vi "Snap.vi"(5 "State In":T1, 7 "Low/Tiny":bool, 8 "error in (no error)":errorcluster, 10 "IMAQ Refs Dani":T3) -> (0 "error out":errorcluster, 1 "Objects":T2[](array[typedef]) {"Aspect Ratio" format="%.2f"; "Orientation" format="%.2f"; "Area" format="%.2f"; "Object Center"."Y" format="%.2f"; "Object Center"."X" format="%.2f"})   [LabVIEW 2015]
uses:
  TypeDefs Host/IMAQ Refs.ctl
  <vilib>/vision/Image Controls.llb/IMAQ Image.ctl
  TypeDefs Host/Object Info.ctl
  TypeDefs Host/States.ctl
  TypeDefs Host/Counter FGV Enum.ctl
  TypeDefs Host/Open Audio FGV Enum.ctl
  <vilib>/vision/NI_Vision_Development_Module.lvlib
panel:
  out "Elapsed time (ms)":u32
  out "Number of Objects":i32
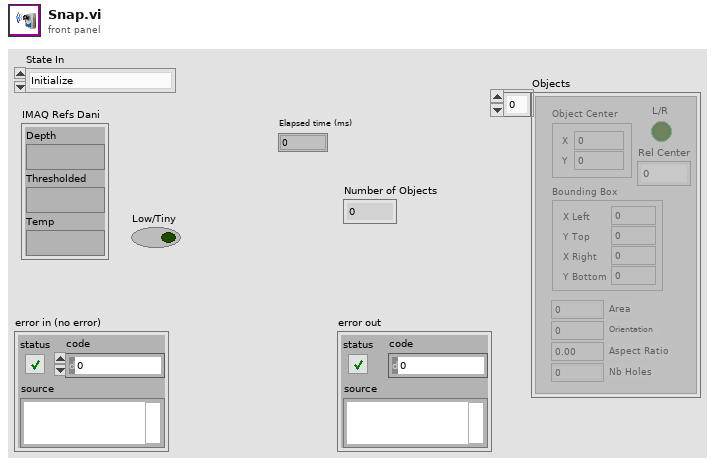
[diagram p1: front panel]
types:
  T1 = typedef "States.ctl" = enum16{"Initialize", "Calibrate", "Create", "Settings", "Shutdown"}
  T2 = typedef "Object Info.ctl" = cluster{"Object Center":cluster{"X":u16, "Y":u16}, "Bounding Box":cluster{"X Left":u16, "Y Top":u16, "X Right":u16, "Y Bottom":u16}, "Area":u16, "Orientation":u16, "Aspect Ratio":sgl, "Nb Holes":u16, "L/R":bool, "Rel Center":u16}
  T3 = typedef "IMAQ Refs.ctl" = cluster{"Thresholded":T4, "Temp":T4, "Depth":T4}
  T4 = typedef "IMAQ Image.ctl" = refnum<image>
  T5 = typedef "Counter FGV Enum.ctl" = enum16{"Get Count", "Set Count"}
  T6 = cluster{"Objects":u16, "Threshold":i32, "Reject Border":bool, "Fill Holes":bool, "Min Object Size":bool, "Min Size":i32, "Max Object Size":bool, "Max Size":i32, "Show Search Area":bool, "Show Center":bool, "Show Bounding Box":bool}
  T7 = typedef "Open Audio FGV Enum.ctl" = enum16{"Get", "Set"}
  T8 = typedef "IMAQ Rectangle" = cluster{"Left":i32, "Top":i32, "Right":i32, "Bottom":i32, "Rotation":dbl}
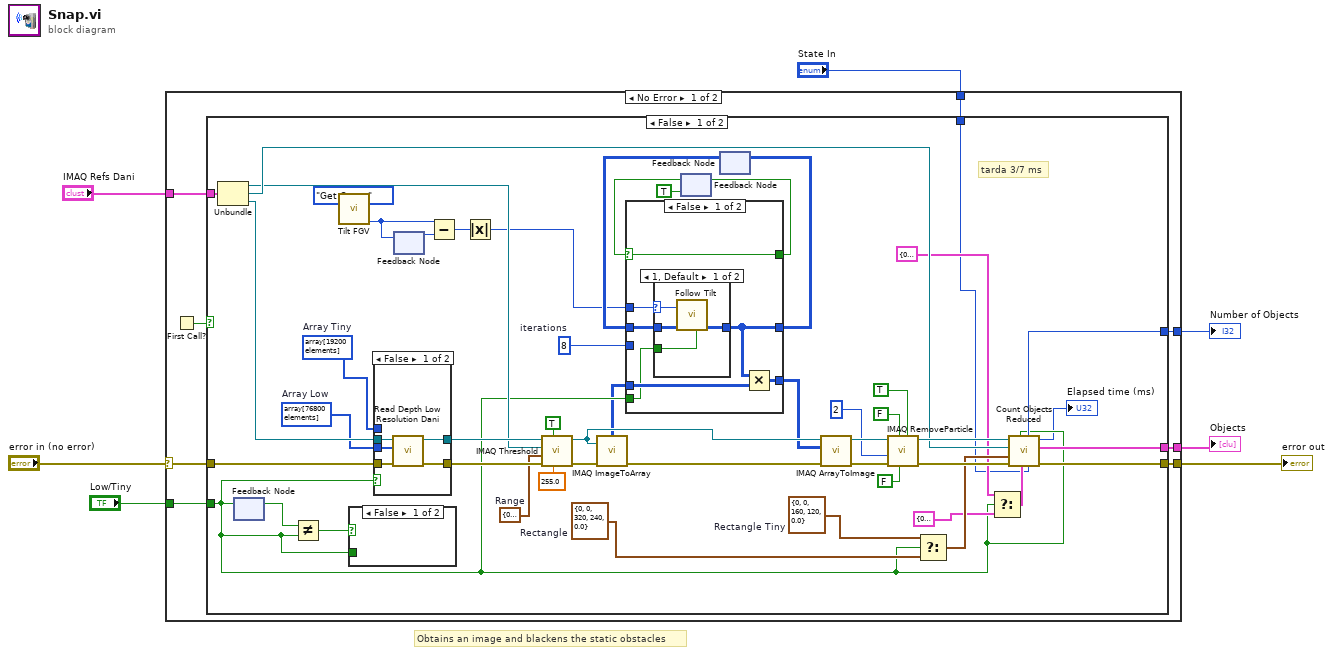
[diagram p0: block diagram]
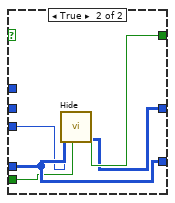
[diagram p3: hidden frame]
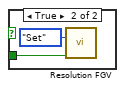
[diagram p4: hidden frame]
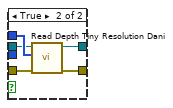
[diagram p5: hidden frame]
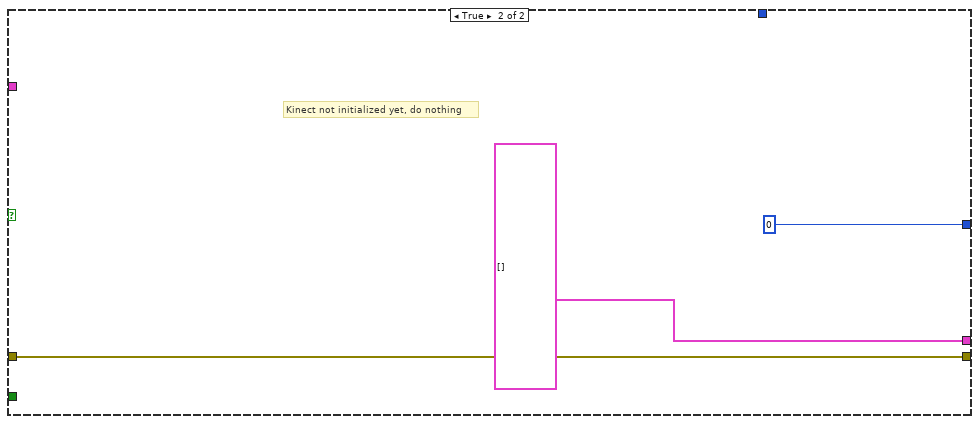
[diagram p6: hidden frame]
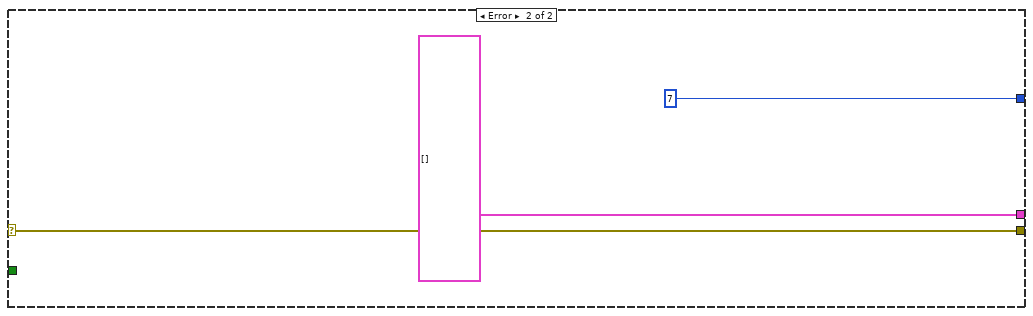
[diagram p7: hidden frame]
diagram:
  # "Obtains an image and blackens the static obstacles"
  n1 = case shown="No Error" "error in (no error)" {
    selector: "error in (no error)" -> [w15 w100]
    tunnel: "IMAQ Refs Dani" -> [w14 _]
    tunnel: [w13 w100] -> w5
    tunnel: [w12 T2[] [] ("Objects")] -> w4
    tunnel: [w11 7 ("Number of Objects")] -> w3
    tunnel: "Low/Tiny" -> [w9 _]
    tunnel: "State In" -> [w8 _]
    frame No Error {
      n2 = First Call?() -> (First Call?: T/F=w10:bool)
      n3 = case shown="False" w10 {
        tunnel: w15 -> [w62 w96]
        tunnel: w14 -> [w61 _]
        tunnel: [w49 w96] -> w13
        tunnel: [w48 T2[] [] ("Objects")] -> w12
        tunnel: [w47 0 ("Number of Objects")] -> w11
        tunnel: w9 -> [w36 _]
        tunnel: w8 -> [w18 _]
        frame False {
          w23 = 8  # iterations
          w44 = T8 {"Left"=0, "Top"=0, "Right"=320, "Bottom"=240, "Rotation"=0.0}  # Rectangle
          w45 = u16[] array[19200 elements]  # Array Tiny
          w43 = T8 {"Left"=0, "Top"=0, "Right"=160, "Bottom"=120, "Rotation"=0.0}  # Rectangle Tiny
          w56 = u16[] array[76800 elements]  # Array Low
          w60 = cluster{"Lower value":sgl, "Upper value":sgl} {"Lower value"=0.0, "Upper value"=151.0}  # Range
          # "tarda 3/7 ms"
          n4 = Unbundle(w61) -> ("Thresholded"=w46:T4, "Temp"=w50:T4, "Depth"=w58:T4)
          n5 = feedback-in #1(w36) -> ()
          n6 = feedback #1() -> (w38:bool)  [unwired: 1 in]
          n7 = Not Equal?(x=w38, y=w36) -> (x != y?=w37:bool)
          n8 = call "Tilt FGV.vi"("Exit FGV Command"=Counter_FGV_Enum."Get Count") -> ("Tilt Out"=w21:i16)  [unwired: 10 in]
          n9 = case shown="False" w37 {
            tunnel: w36 -> [_ w83]
            frame False {
            }
            frame True {
              n10 = call "Resolution FGV.vi"("Command"=Open_Audio_FGV_Enum."Set", "L/T"=w83) -> ()  [unwired: 9 in, 1 out]
            }
          }
          n11 = case shown="False" w36 {
            tunnel: [w89 w94] -> w65
            tunnel: w62 -> [w88 w91]
            tunnel: [w87 w90] -> w59
            tunnel: w58 -> [w86 w92]
            tunnel: w56 -> [w85 _]
            tunnel: w45 -> [_ w93]
            frame False {
              n12 = call "Read Depth Low Resolution Dani.vi"("error in (no error)"=w88, "depth"=w85, "Image In"=w86) -> ("error out"=w89:errorcluster, "Image Out"=w87:T4)  [unwired: 7 in]
            }
            frame True {
              n13 = call "Read Depth Tiny Resolution Dani.vi"("error in (no error)"=w91, "depth"=w93, "Image In"=w92) -> ("error out"=w94:errorcluster, "Image Out"=w90:T4)  [unwired: 7 in]
            }
          }
          n14 = feedback #2() -> (w20:i16)  [unwired: 1 in]
          n15 = feedback-in #2(w21) -> ()
          n16 = Subtract(x=w21, y=w20) -> (x-y=w17:i16)
          n17 = Absolute Value(x=w17) -> (abs(x)=w16:i16)
          n18 = call "IMAQ Threshold"("Replace Value"=sgl 255.0, "Keep/Replace Value (Replace)"=TRUE, "error in (no error)"=w65, "Range"=w60, "Image Dst"=w46, "Image Src"=w59) -> ("error out"=w57:errorcluster, "Image Dst Out"=w55:T4)  [unwired: 4 in]
          n19 = call "IMAQ ImageToArray"("error in (no error)"=w57, "Image"=w55) -> ("error out"=w30:errorcluster, "Image Pixels (U8)"=w31:u8[][])  [unwired: 2 in, 3 out]
          n20 = feedback #3(TRUE ("finish")) -> (w28:bool)
          n21 = feedback #4() -> (w25:u8[][])  [unwired: 1 in]
          n22 = case shown="False" w28 {
            selector: w28 -> [w72 _]
            tunnel: w36 -> [w66 w78]
            tunnel: [w72 w82] -> w24
            tunnel: w31 -> [w71 w81]
            tunnel: [w70 w81] -> w29
            tunnel: [w68 w80] -> w26
            tunnel: w25 -> [w67 _]
            tunnel: w23 -> [_ w79]
            tunnel: w16 -> [w69 _]
            frame False {
              n23 = case shown="1, Default" w69 {
                selector: w69 -> [w74 _]
                tunnel: [w75 w77] -> w68
                tunnel: w67 -> [w76 w77]
                tunnel: w66 -> [w73 _]
                frame 1, Default {
                  n24 = call "Follow Tilt.vi"("L/T"=w73, "deg"=w74, "In"=w76) -> ("Out"=w75:u8[][])  [unwired: 8 in]
                }
                frame 0 {
                }
              }
              n25 = Multiply(x=w68, y=w71) -> (x*y=w70:u8[][])
            }
            frame True {
              n26 = call "Hide.vi"("L/T"=w78, "iterations"=w79, "Image Pixels In (U8)"=w81) -> ("static"=w80:u8[][], "hide"=w82:bool)  [unwired: 7 in]
            }
          }
          n27 = feedback-in #3(w24) -> ()
          n28 = feedback-in #4(w26) -> ()
          n29 = call "IMAQ ArrayToImage"("error in (no error)"=w30, "Image Pixels (U8)"=w29, "Image"=w55) -> ("error out"=w54:errorcluster, "Image Out"=w53:T4)  [unwired: 7 in]
          n30 = call "IMAQ RemoveParticle"("Connectivity 4/8 (8)"=TRUE, "Low Pass/High Pass (Low)"=FALSE, "Square/Hexa (Square)"=FALSE, "error in (no error)"=w54, "Number of Erosion"=2, "Image Src"=w53) -> ("error out"=w51:errorcluster, "Image Dst Out"=w52:T4)  [unwired: 4 in]
          n31 = Select(t=w43, s=w36, f=w44) -> (s? t:f=w42:T8)
          n32 = Select(t=T6 {"Objects"=0, "Threshold"=254, "Reject Border"=TRUE, "Fill Holes"=FALSE, "Min Object Size"=FALSE, "Min Size"=25, "Max Object Size"=TRUE, "Max Size"=500, "Show Search Area"=TRUE, "Show Center"=FALSE, "Show Bounding Box"=TRUE} ("Settings"), s=w36, f=T6 {"Objects"=0, "Threshold"=254, "Reject Border"=TRUE, "Fill Holes"=FALSE, "Min Object Size"=FALSE, "Min Size"=100, "Max Object Size"=TRUE, "Max Size"=2000, "Show Search Area"=TRUE, "Show Center"=FALSE, "Show Bounding Box"=TRUE} ("Settings")) -> (s? t:f=w39:T6)
          n33 = call "Count Objects Reduced.vi"("State In"=w18, "Settings"=w39, "Low/Tiny"=w36, "error in"=w51, "Rectangle"=w42, "Temp"=w50, "Image"=w52) -> ("error out"=w49:errorcluster, "Objects"=w48:T2[], "Elapsed time (ms)"=→"Elapsed time (ms)":u32, "Number of Objects"=w47:i32)  [unwired: 1 in]
        }
        frame True {
          # "Kinect not initialized yet, do nothing"
        }
      }
    }
    frame Error {
    }
  }
  "error out" <- w5
  "Objects" <- w4
  "Number of Objects" <- w3
